vi "Read Channels.vi"(8 "error in (no error)":errorcluster, 11 "Cryo Cooler in":refnum<class "Cryo Cooler.lvclass">) -> (0 "error out":errorcluster, 2 "Channels":string[](array[string]), 3 "Cryo Cooler out":refnum<class "Cryo Cooler.lvclass">)   [LabVIEW 2024, in "Cryo Cooler.lvclass"]
uses:
  Cryo Cooler.lvclass
  Cryo Cooler.lvclass/Cryo Cooler.ctl
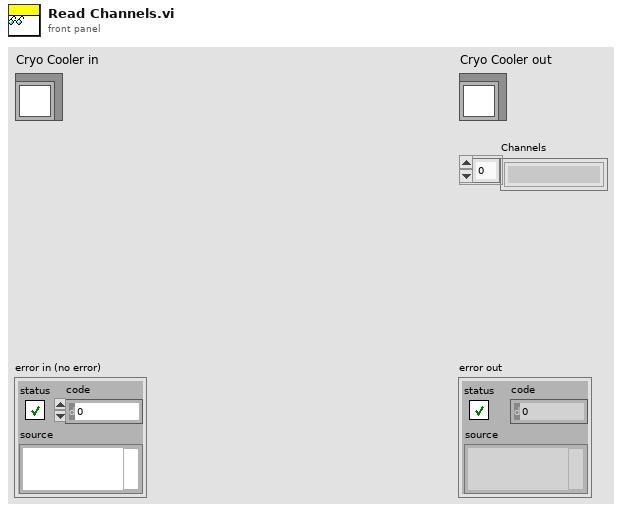
[diagram p1: front panel]
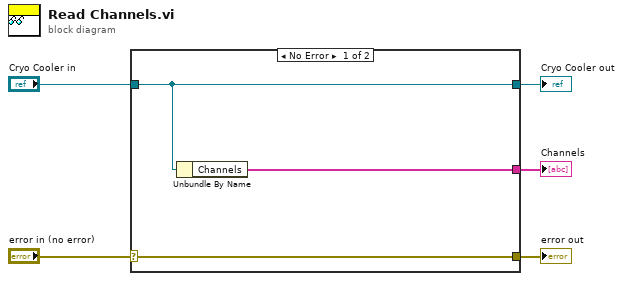
[diagram p0: block diagram]
diagram:
  n1 = case shown="No Error" "error in (no error)" {
    selector: "error in (no error)" -> [w8 w9]
    tunnel: [w8 w9] -> w4
    tunnel: [w7 w10] -> w2
    tunnel: "Cryo Cooler in" -> [w7 w10]
    tunnel: [w6 _] -> w1
    frame No Error {
      n2 = Unbundle By Name(w7) -> ("Channels"=w6:string[])
    }
    frame Error {
    }
  }
  "error out" <- w4
  "Cryo Cooler out" <- w2
  "Channels" <- w1
